vi "processString.vi"(8 "error in (no error)":errorcluster, 10 "Message in":string, 11 "Sent message in":refnum<class "MixerMessage.lvclass">) -> (0 "error out":errorcluster, 1 "found?":bool, 2 "response":T1, 3 "Sent message out":refnum<class "MixerMessage.lvclass">, 4 "isAck?":bool, 5 "Remaining buffer":string)   [LabVIEW 2013, in "MixerMessage.lvclass"]
doc: "Parses and interpretes the input string. If a complete packet from the remote host is found, \"found?\" should return TRUE. In that the case, the response should contain the type and the message data in the variant. \nIf the found message is an acknowledgement to the \"Sent message in\", the isAck? boolean should return TRUE.\nAnything left in the Message in string after the first message has been found should be returned in Remaining buffer"
uses:
  MixerMessage.lvclass
  response.ctl
  driver_status.ctl
  MixerOperation.ctl
  MixerParam.ctl
  Driver/TcpDriver/MixerResponse.ctl
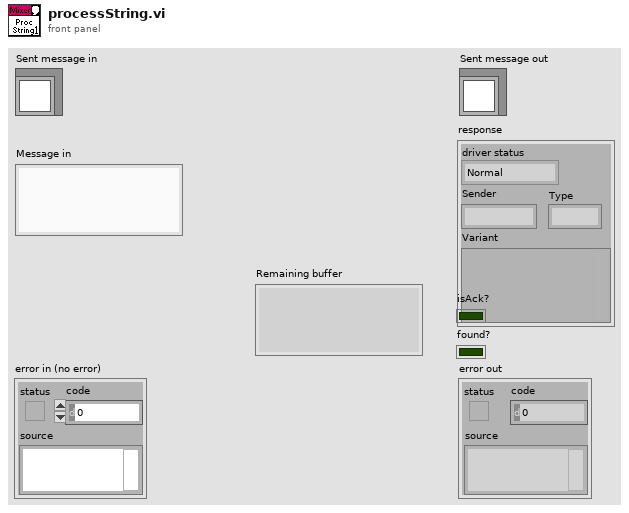
[diagram p1: front panel]
types:
  T1 = typedef "response.ctl" = cluster{"driver status":T2, "Sender":string, "Type":i32, "Variant":variant}
  T2 = typedef "driver_status.ctl" = enum16{"Normal", "Startup", "Connection lost", "Reconnected", "Timeout", "Idle", "Busy"}
  T3 = typedef "MixerResponse.ctl" = cluster{"Operation":T4, "Param":T5, "value":dbl}
  T4 = typedef "MixerMessage.lvclass/MixerOperation.ctl" = enum16{"Get", "Set"}
  T5 = typedef "MixerMessage.lvclass/MixerParam.ctl" = enum16{"a", "b", "fm"}
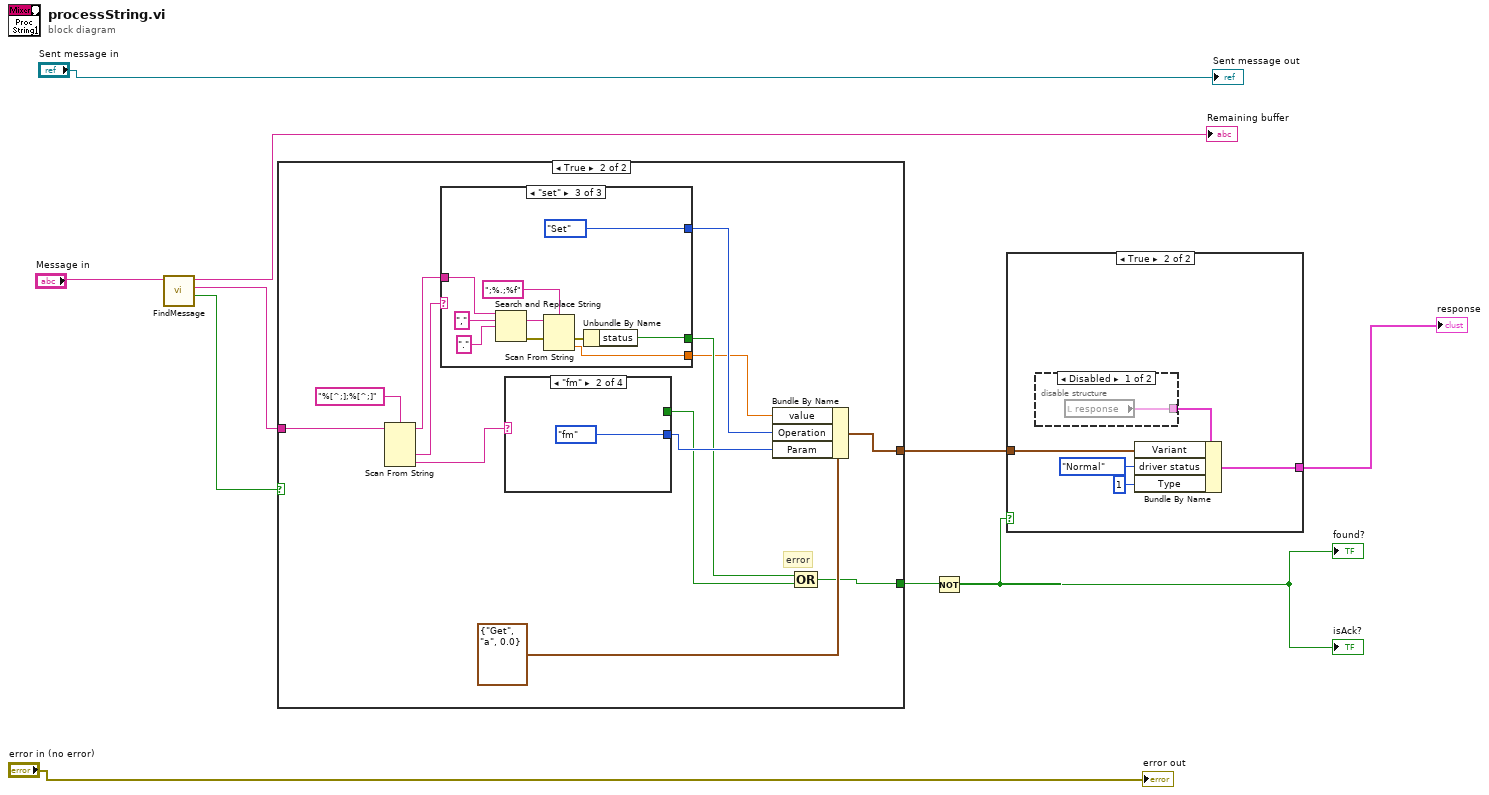
[diagram p0: block diagram]
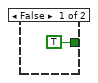
[diagram p4: hidden frame]
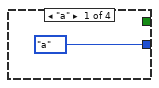
[diagram p5: hidden frame]
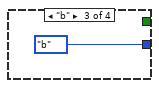
[diagram p6: hidden frame]
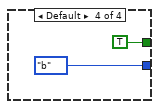
[diagram p7: hidden frame]
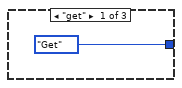
[diagram p8: hidden frame]
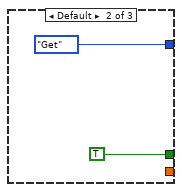
[diagram p9: hidden frame]
diagram:
  n1 = call "FindMessage.vi"("Message in"="Message in") -> ("found?"=w7:bool, "Message"=w8:string, "Remaining buffer"=→"Remaining buffer":string)  [unwired: 8 in]
  n2 = case shown="True" w7 {
    tunnel: w8 -> [_ w24]
    tunnel: [_ w17] -> w2
    tunnel: [TRUE w14] -> w6
    frame False {
    }
    frame True {
      # "error"
      n3 = Scan From String(format string="%[^;];%[^;]", input string=w24) -> (remaining string=w12:string, output 1=w22:string, output 2=w21:string)  [unwired: 4 in, 2 out]
      n4 = case shown="\"set\"" w22 {
        tunnel: [MixerOperation."Get" ("MixerOperation") MixerOperation."Get" ("MixerOperation") MixerOperation."Set" ("MixerOperation")] -> w19
        tunnel: [_ TRUE w34] -> w16
        tunnel: [_ _ w35] -> w13
        tunnel: w12 -> [_ _ w33]
        frame "get" {
        }
        frame Default {
        }
        frame "set" {
          n5 = Search and Replace String(input string=w33, search string=",", replace string="." ("search string")) -> (result string=w39:string, error out=w40:errorcluster)  [unwired: 5 in, 2 out]
          n6 = Scan From String(format string=";%.;%f", input string=w39, error in=w40) -> (error out=w36:errorcluster, output 1=w35:dbl)  [unwired: 2 in, 2 out]
          n7 = Unbundle By Name(w36) -> ("status"=w34:bool)
        }
      }
      n8 = case shown="\"fm\"" w21 {
        tunnel: [MixerParam."a" ("MixerParam") MixerParam."fm" ("MixerParam") MixerParam."b" ("MixerParam") MixerParam."b" ("MixerParam")] -> w18
        tunnel: [_ _ _ TRUE] -> w15
        frame "a" {
        }
        frame "fm" {
        }
        frame "b" {
        }
        frame Default {
        }
      }
      n9 = Bundle By Name(cluster=T3 {"Operation"=enum."Get", "Param"=enum."a", "value"=0.0} ("MixerRespone"), "value"=w13, "Operation"=w19, "Param"=w18) -> (w17:T3)
      n10 = Compound Arithmetic op=OR(w16, w15) -> (w14:bool)
    }
  }
  n11 = Not(x=w6) -> (.not. x?=w3:bool)
  "isAck?" <- w3
  "found?" <- w3
  n12 = case shown="True" w3 {
    tunnel: w2 -> [_ w44]
    tunnel: [_ w43] -> w1
    frame False {
    }
    frame True {
      n13 = disable-structure shown="Disabled" {
        disable-tunnel: [w48 _] -> w47
        frame Disabled {
          n14 = local read "response"() -> (w48:T1)
        }
        frame Enabled {
        }
      }
      n15 = Bundle By Name(cluster=w47, "Variant"=w44, "driver status"=driver_status."Normal", "Type"=1) -> (w43:T1)
    }
  }
  "response" <- w1
  "error out" <- "error in (no error)"
  "Sent message out" <- "Sent message in"
